vi "Set VI Icon Text Layer.vi"(10 "Text":T1={"Line 1 text"="", "Line 2 text"="a", "Line 3 text"="b", "Line 4 text"="c"}, 11 "VI in":refnum<vi>) -> (0 "error out":errorcluster, 3 "VI out":refnum<vi>)   [LabVIEW 2019, in "gRPC Template Creation Utility.lvlib"]
doc: "This example reads the current icon of a VI and updates it with an entirely new icon which primarily focuses on the Text Layer."
uses:
  gRPC Template Creation Utility.lvlib
  <vilib>/LabVIEW Icon API/LabVIEW Icon API.lvlib
  <vilib>/LabVIEW Icon API/API_Text.ctl
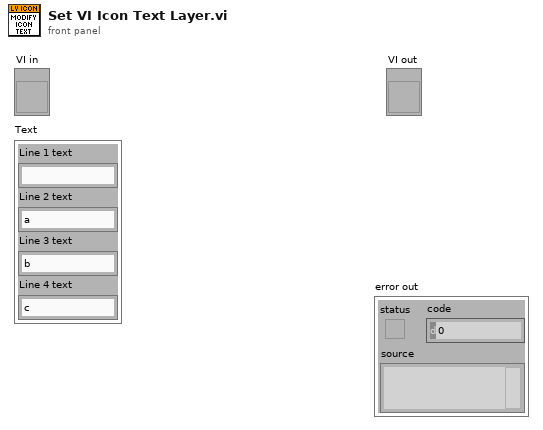
[diagram p1: front panel]
types:
  T1 = typedef "LabVIEW Icon API.lvlib/API_Text.ctl" = cluster{"Line 1 text":string, "Line 2 text":string, "Line 3 text":string, "Line 4 text":string}
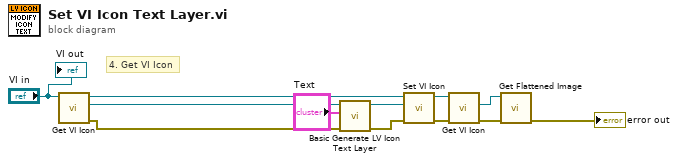
[diagram p0: block diagram]
diagram:
  # "4. Get VI Icon"
  n1 = call <vilib>:"Get VI Icon.vi"("VI Refnum in"="VI in") -> ("error out"=w2:errorcluster, "Icon"=w3:refnum<class "Icon.lvclass">, "VI Refnum out"=w12:refnum<vi>)  [unwired: 8 in]
  n2 = call "Basic Generate LV Icon Text Layer.vi"("error in (no error)"=w2, "Text"="Text", "Icon"=w3) -> ("error out"=w11:errorcluster, "Icon.lvlclass out"=w10:refnum<class "Icon.lvclass">)  [unwired: 7 in]
  n3 = call <vilib>:"Set VI Icon.vi"("error in (no error)"=w11, "Icon"=w10, "VI Refnum in"=w12) -> ("error out"=w9:errorcluster, "VI Refnum out"=w8:refnum<vi>)  [unwired: 7 in]
  n4 = call <vilib>:"Get VI Icon.vi"("error in (no error)"=w9, "VI Refnum in"=w8) -> ("error out"=w7:errorcluster, "Icon"=w6:refnum<class "Icon.lvclass">)  [unwired: 7 in, 1 out]
  n5 = call <vilib>:"Get Flattened Image.vi"("error in (no error)"=w7, "lv_icon.lvlib:Icon.lvclass in"=w6) -> ("error out"=→"error out":errorcluster)  [unwired: 6 in, 3 out]
  "VI out" <- "VI in"
